vi "Choose_Panels.vi"(11 "Array":string[](array[string])) -> (3 "Array 2":string[](array[string]))   [LabVIEW 2018]
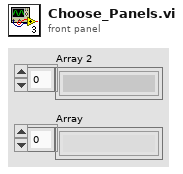
[diagram p1: front panel]
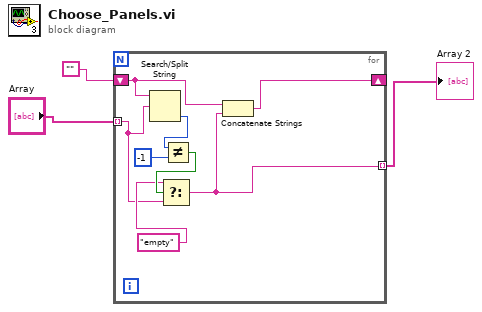
[diagram p0: block diagram]
diagram:
  n1 = for {
    tunnel: "Array" -> [w4] mode=indexing
    shift-right: [w5] -> _
    shift-left: "" -> [w7]
    tunnel: [w6] -> w1 mode=indexing
    n2 = Search/Split String(string=w7, search string/char (-)=w4) -> (offset of match=w11:i32)  [unwired: 1 in, 2 out]
    n3 = Not Equal?(x=w11, y=-1) -> (x != y?=w9:bool)
    n4 = Select(t="empty", s=w9, f=w4) -> (s? t:f=w6:string)
    n5 = Concatenate Strings(w7, w6) -> (w5:string)
  }
  "Array 2" <- w1
